vi "user32_SetWindowPos.vi"(8 "error in (no error)":errorcluster, 9 "uFlags":u32, 10 "hWndInsertAfter":i64, 11 "hWnd":i64) -> (0 "error out":errorcluster, 3 "return":i32)   [LabVIEW 2020]
uses:
  user32.dll
panel:
  in  "cy":i32
  in  "cx":i32
  in  "Y":i32
  in  "X":i32
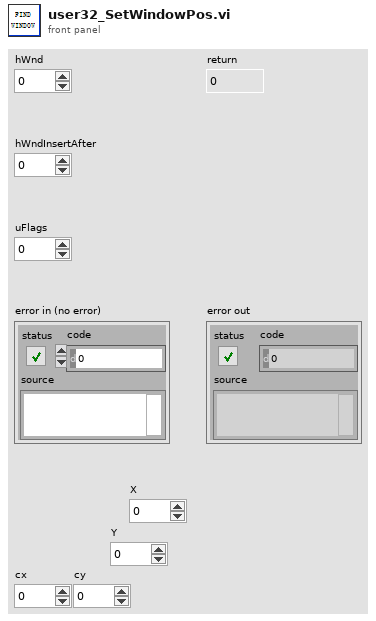
[diagram p1: front panel]
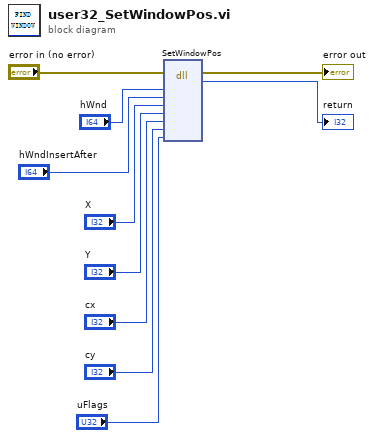
[diagram p0: block diagram]
diagram:
  n1 = dll-call lib="user32.dll" fn="SetWindowPos"(error in="error in (no error)", "hWnd"="hWnd", "hWndInsertAfter"="hWndInsertAfter", "X"="X", "Y"="Y", "cx"="cx", "cy"="cy", "uFlags"="uFlags") -> (error out=→"error out":errorcluster, "返回值"=→"return":i32)  [unwired: 9 in, 1 out]
